vi "Panel Split Engine.vi"() -> ()   [LabVIEW 2013]
uses:
  PanelRootNode.lvclass
  <vilib>/Utility/error.llb/DialogType.ctl
  share/QueueManager.llb/Destroy.vi
  share/QueueManager.llb/CreatQueue.vi
  share/QueueManager.llb/Remove.vi
  PanelLinkNode/PanelLinkNode.lvclass
  PanelDataNode/PanelDataNode.lvclass
panel:
  out "SelfNode*":refnum<data-value>
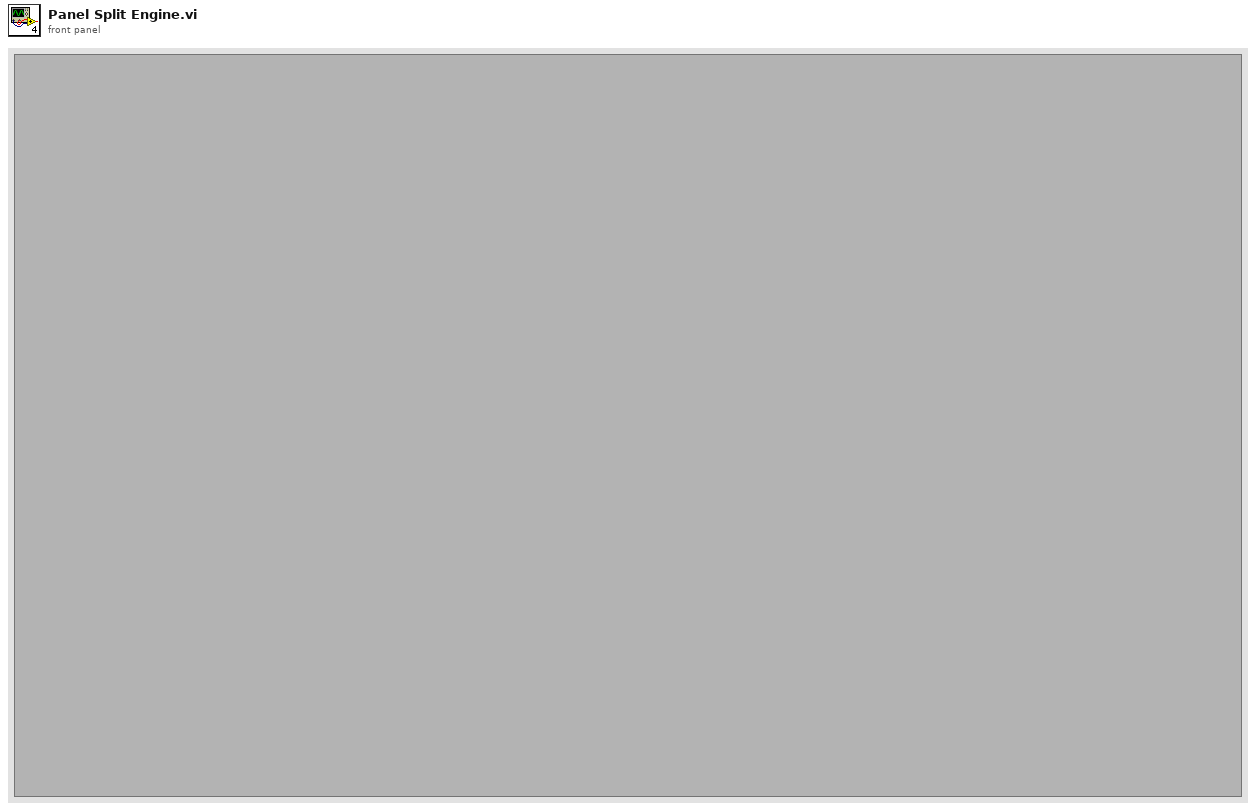
[diagram p1: front panel]
types:
  T1 = cluster{"error":errorcluster, "Event":string, "Data":variant, "Q_Local":string, "RootNode*":refnum<data-value>, "Caller":string}
  T2 = typedef "DialogType.ctl" = u16
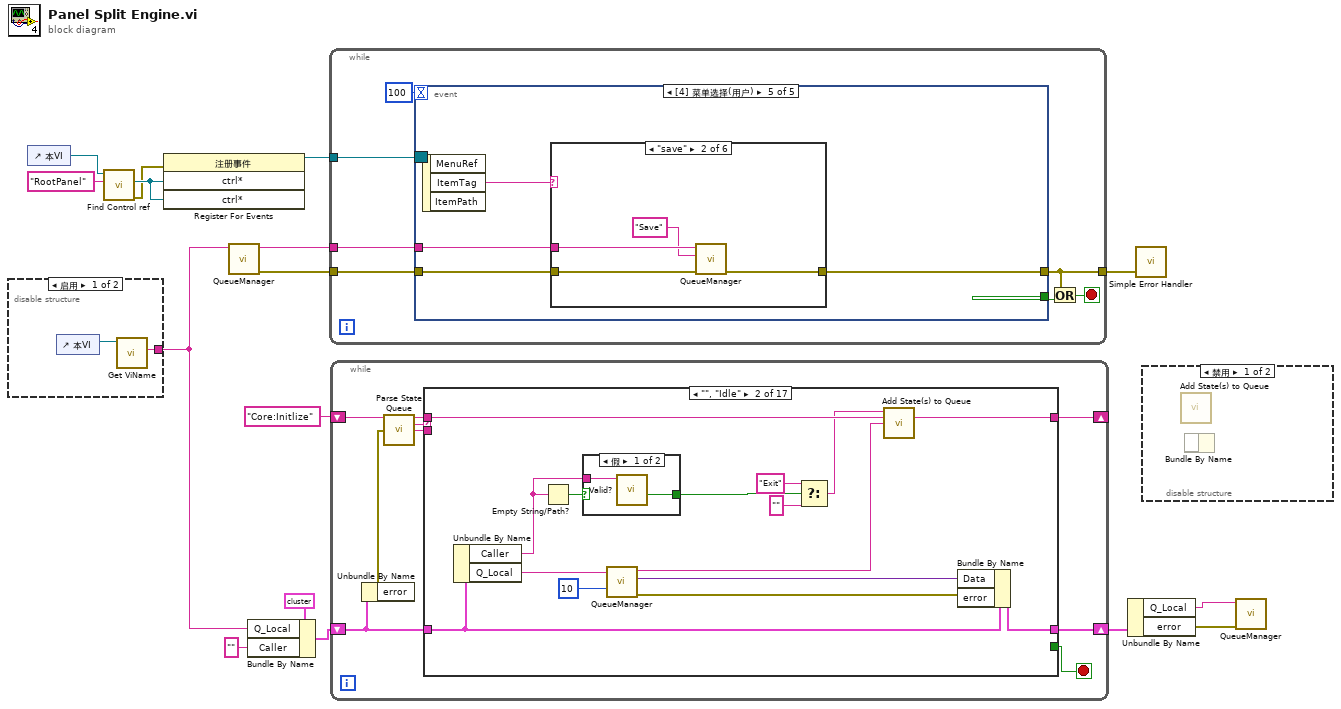
[diagram p0: block diagram]
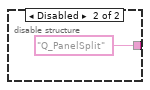
[diagram p2: hidden frame]
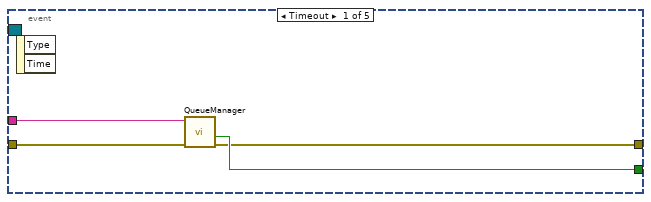
[diagram p4: hidden frame]
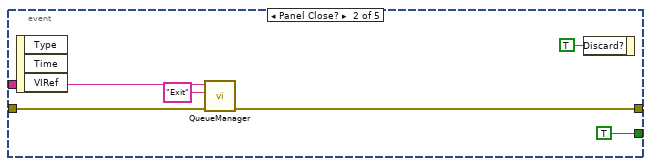
[diagram p5: hidden frame]
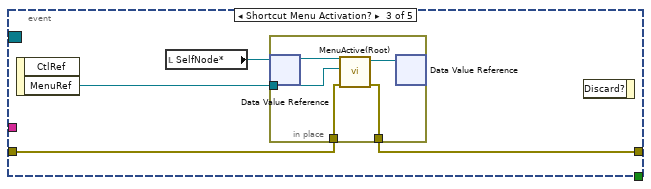
[diagram p6: hidden frame]
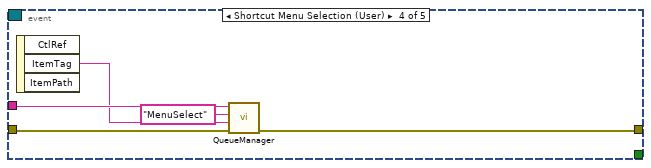
[diagram p7: hidden frame]
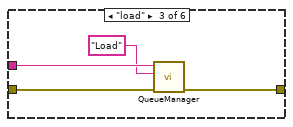
[diagram p9: hidden frame]
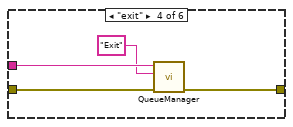
[diagram p10: hidden frame]
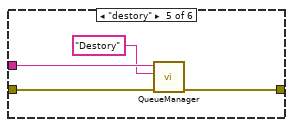
[diagram p11: hidden frame]
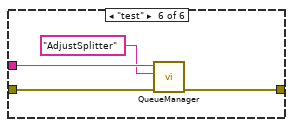
[diagram p12: hidden frame]
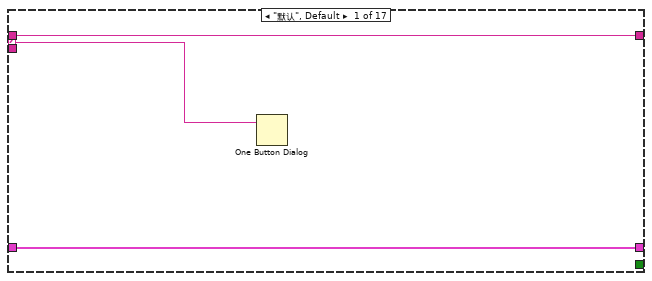
[diagram p13: hidden frame]
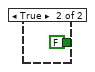
[diagram p14: hidden frame]
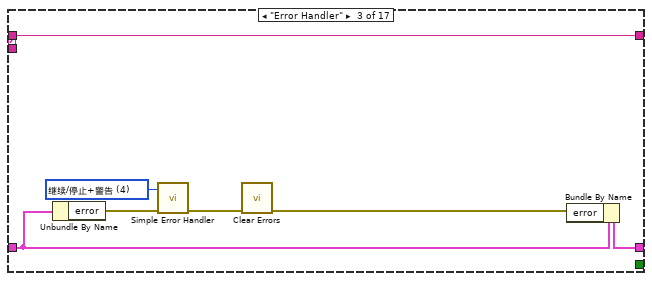
[diagram p15: hidden frame]
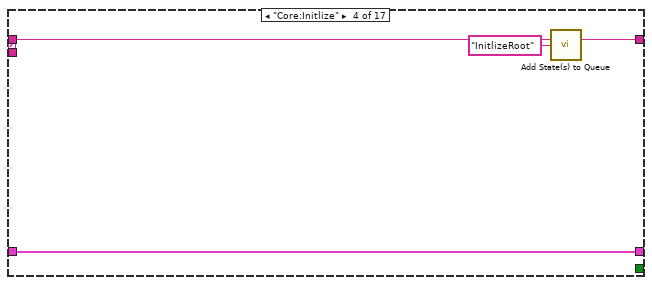
[diagram p16: hidden frame]
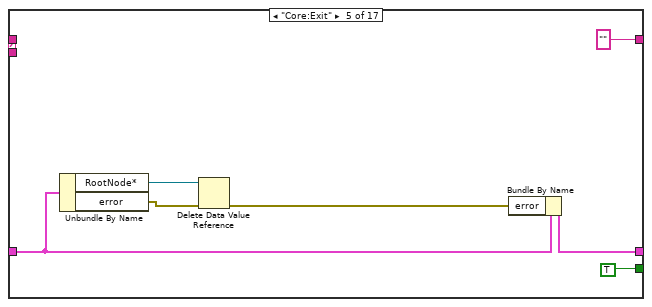
[diagram p17: hidden frame]
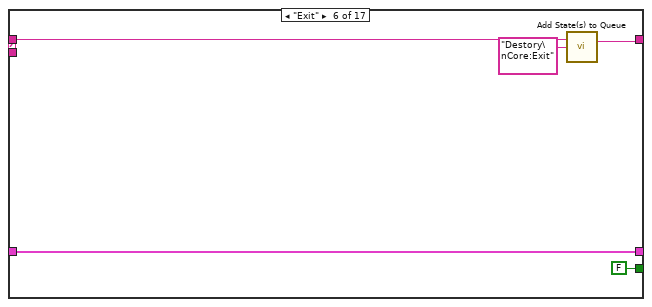
[diagram p18: hidden frame]
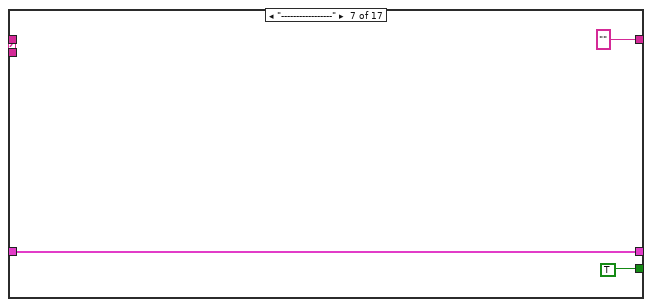
[diagram p19: hidden frame]
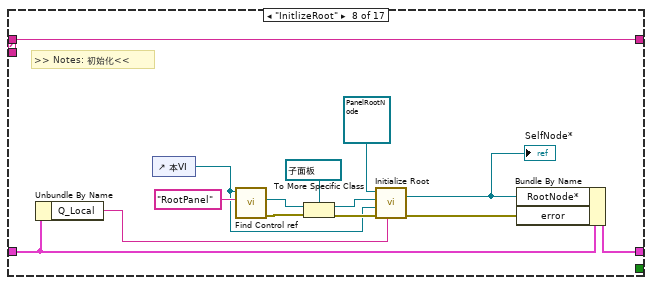
[diagram p20: hidden frame]
diagram:
  n1 = disable-structure shown="启用" {
    disable-tunnel: [w16 "Q_PanelSplit" ("QueueName")] -> w3
    frame Enabled {
      n2 = control-ref of="本VI"() -> (w17:refnum<vi>)
      n3 = call "Get ViName.vi"("VI*"=w17) -> ("VI Name"=w16:string)  [unwired: 8 in, 2 out]
    }
    frame Disabled {
    }
  }
  n4 = control-ref of="本VI"() -> (w7:refnum<vi>)
  n5 = call "Find Control ref.vi"("control name"="RootPanel", "panelvi*"=w7) -> ("error out"=w2:errorcluster, "ctrl*"=w5:refnum<vi>)  [unwired: 7 in, 1 out]
  n6 = register-events(error in=w2, w5, w5) -> (reference out=w4:refnum<event-registration>)  [unwired: 1 in, 1 out]
  n7 = call-poly "QueueManager.vi"("QueueName"=w3) -> ("error out"=w15:errorcluster)  [unwired: 10 in]
  n8 = Bundle By Name(cluster=T1 {"error"={"status"=FALSE, "code"=0, "source"=""}, "Event"="", "Data"=variant, "Q_Local"="", "RootNode*"=refnum, "Caller"=""} ("TmpData"), "Q_Local"=w3, "Caller"="") -> (w9:T1)
  n9 = while {
    tunnel: w15 -> [w24]
    tunnel: w3 -> [w25]
    tunnel: [w21] -> w11
    tunnel: w4 -> [w19]
    stop <- w22 stop-if-true
    n10 = event shown="[4] 菜单选择(用户)" {
      selector: w19 -> [_ _ _ _ _]
      dyn-events: _ -> [_ _ _ _ _]
      timeout: 100 -> [_ _ _ _ _]
      tunnel: [w27 TRUE _ _ _] -> w23
      tunnel: w25 -> [w29 w34 _ w49 w52]
      tunnel: w24 -> [w28 w33 w38 w48 w51]
      tunnel: [w26 w32 w39 w47 w50] -> w21
      event Timeout {
        n11 = event-data() -> ()  [unwired: 1 in, 2 out]
        n12 = call-poly "QueueManager.vi"("error in (no error)"=w28, "Queue Name(unamed)"=w29) -> ("error out"=w26:errorcluster, "Not Exist?"=w27:bool)  [unwired: 8 in]
      }
      event Panel Close? {
        n13 = event-data() -> ()  [unwired: 1 in, 3 out]
        n14 = call-poly "QueueManager.vi"("error in"=w33, "Event"="Exit", "QueueName"=w34) -> ("error out"=w32:errorcluster)  [unwired: 7 in, 1 out]
        n15 = event-data("Discard?"=TRUE ("放弃？")) -> ()  [unwired: 1 in, 1 out]
      }
      event Shortcut Menu Activation? {
        n16 = event-data() -> ("MenuRef"=w37:refnum<k9>)  [unwired: 1 in, 1 out]
        n17 = local read "SelfNode*"() -> (w36:refnum<data-value>)
        n18 = in-place {
          in-place-border: w37 -> [w42]
          in-place-border: w38 -> [w41]
          in-place-border: [w40] -> w39
          n19 = in-place-dvr #1(w36) -> (w44:refnum<class "PanelRootNode.lvclass">)  [unwired: 1 out]
          n20 = call "MenuActive(Root).vi"("error in (no error)"=w41, "菜单引用"=w42, "PanelDataNode 输入"=w44) -> ("error out"=w40:errorcluster, "PanelDataNode 输出"=w43:refnum<class "PanelRootNode.lvclass">)  [unwired: 7 in]
          n21 = in-place-dvr #1(w43) -> ()  [unwired: 2 out]
        }
        n22 = event-data() -> ()  [unwired: 2 in, 1 out]
      }
      event Shortcut Menu Selection (User) {
        n23 = event-data() -> ("ItemTag"=w46:string)  [unwired: 1 in, 2 out]
        n24 = call-poly "QueueManager.vi"("error in"=w48, "Data"=w46, "Event"="MenuSelect", "QueueName"=w49) -> ("error out"=w47:errorcluster)  [unwired: 6 in, 1 out]
      }
      event Menu Selection (User) {
        n25 = event-data() -> ("ItemTag"=w53:string)  [unwired: 1 in, 2 out]
        n26 = case shown="\"save\"" w53 {
          tunnel: w52 -> [_ w58 w62 w66 w70 w74]
          tunnel: w51 -> [w54 w56 w60 w64 w68 w72]
          tunnel: [w54 w55 w59 w63 w67 w71] -> w50
          frame "假", Default {
          }
          frame "save" {
            n27 = call-poly "QueueManager.vi"("error in"=w56, "Event"="Save", "QueueName"=w58) -> ("error out"=w55:errorcluster)  [unwired: 7 in, 1 out]
          }
          frame "load" {
            n28 = call-poly "QueueManager.vi"("error in"=w60, "Event"="Load", "QueueName"=w62) -> ("error out"=w59:errorcluster)  [unwired: 7 in, 1 out]
          }
          frame "exit" {
            n29 = call-poly "QueueManager.vi"("error in"=w64, "Event"="Exit", "QueueName"=w66) -> ("error out"=w63:errorcluster)  [unwired: 7 in, 1 out]
          }
          frame "destory" {
            n30 = call-poly "QueueManager.vi"("error in"=w68, "Event"="Destory", "QueueName"=w70) -> ("error out"=w67:errorcluster)  [unwired: 7 in, 1 out]
          }
          frame "test" {
            n31 = call-poly "QueueManager.vi"("error in"=w72, "Event"="AdjustSplitter", "QueueName"=w74) -> ("error out"=w71:errorcluster)  [unwired: 7 in, 1 out]
          }
        }
      }
    }
    n32 = Or(x=w21, y=w23) -> (x .or. y?=w22:bool)
  }
  n33 = while {
    shift-right: [w76] -> w12
    shift-left: w9 -> [w77]
    shift-right: [w75] -> _
    shift-left: "Core:Initlize" -> [w83]
    stop <- w79 stop-if-true
    n34 = Unbundle By Name(w77) -> ("error"=w78:errorcluster)
    n35 = call "Parse State Queue.vi"("State Queue"=w83, "Error In (no error)"=w78) -> ("Remaining States"=w82:string, "Current State"=w81:string, "Arguments"=w80:string)  [unwired: 10 in, 1 out]
    n36 = case shown="\"\", \"Idle\"" w81 {
      selector: w81 -> [w84 _ _ _ _ _ _ _ _ _ _ _ _ _ _ _ _]
      tunnel: w82 -> [w85 w97 w111 w114 _ w127 _ w144 w150 w166 w176 w191 w201 w211 w221 w230 w245]
      tunnel: w80 -> [_ _ _ _ _ _ _ _ _ _ _ _ _ _ _ _ _]
      tunnel: [_ _ _ _ TRUE FALSE TRUE _ _ _ _ _ _ _ _ _ _] -> w79
      tunnel: w77 -> [w86 w94 w107 w115 w118 w124 w129 w132 w152 w164 w180 w190 w199 w209 w219 w228 w243]
      tunnel: [w86 w100 w106 w115 w117 w124 w129 w135 w151 w163 w179 w189 w198 w208 w218 w227 w242] -> w76
      tunnel: [w85 w96 w111 w113 "" ("Remaining States") w126 "" ("Remaining States") w144 w150 w166 w175 w191 w201 w211 w221 w230 w245] -> w75
      frame "默认", Default {
        n37 = One Button Dialog(message=w84) -> ()  [unwired: 1 in, 1 out]
      }
      frame "", "Idle" {
        n38 = Unbundle By Name(w94) -> ("Caller"=w88:string, "Q_Local"=w93:string)
        n39 = Empty String/Path?(string/path=w88) -> (empty?=w92:bool)
        n40 = case shown="假" w92 {
          tunnel: [w103 FALSE ("Not Exist?")] -> w91
          tunnel: w88 -> [w102 _]
          frame False {
            n41 = call "Valid?.vi"("Queue Name(unamed)"=w102) -> ("Not Exist?"=w103:bool)  [unwired: 9 in, 1 out]
          }
          frame True {
          }
        }
        n42 = call-poly "QueueManager.vi"("Time out(-1)"=10, "Queue Name"=w93) -> ("error out"=w101:errorcluster, "Data"=w99:variant, "Event"=w98:string)  [unwired: 6 in, 1 out]
        n43 = Select(t="Exit" ("Event"), s=w91, f="") -> (s? t:f=w87:string)
        n44 = call "Add State(s) to Queue.vi"("State(s) in Front (\"\")"=w87, "State(s) in (\"\")"=w97, "State(s) at Back (\"\")"=w98) -> ("States Out"=w96:string)  [unwired: 12 in]
        n45 = Bundle By Name(cluster=w94, "Data"=w99, "error"=w101) -> (w100:T1)
      }
      frame "Error Handler" {
        w105 = T2 4 items=["无对话框", "确定信息", "继续或停止信息", "确定信息＋警告", "继续/停止+警告"] ("type of dialog (OK msg:1)")
        n46 = Unbundle By Name(w107) -> ("error"=w108:errorcluster)
        n47 = call <vilib>:"Simple Error Handler.vi"("type of dialog (OK msg:1)"=w105, "error in (no error)"=w108) -> ("error out"=w109:errorcluster)  [unwired: 3 in, 4 out]
        n48 = call <vilib>:"Clear Errors.vi"("error in (no error)"=w109) -> ("error out"=w110:errorcluster)  [unwired: 6 in]
        n49 = Bundle By Name(cluster=w107, "error"=w110) -> (w106:T1)
      }
      frame "Core:Initlize" {
        n50 = call "Add State(s) to Queue.vi"("State(s) in (\"\")"=w114, "State(s) at Back (\"\")"="InitlizeRoot" ("State(s) at Back (\"\")")) -> ("States Out"=w113:string)  [unwired: 13 in]
      }
      frame "Core:Exit" {
        n51 = Unbundle By Name(w118) -> ("RootNode*"=w120:refnum<data-value>, "error"=w116:errorcluster)
        n52 = Delete Data Value Reference(data value reference=w120, error in=w116) -> (error out=w119:errorcluster)  [unwired: 1 out]
        n53 = Bundle By Name(cluster=w118, "error"=w119) -> (w117:T1)
      }
      frame "Exit" {
        n54 = call "Add State(s) to Queue.vi"("State(s) in (\"\")"=w127, "State(s) at Back (\"\")"="Destory\nCore:Exit" ("State(s) at Back (\"\")")) -> ("States Out"=w126:string)  [unwired: 13 in]
      }
      frame "-----------------" {
      }
      frame "InitlizeRoot" {
        # ">> Notes: 初始化<<"
        n55 = Unbundle By Name(w132) -> ("Q_Local"=w131:string)
        n56 = control-ref of="本VI"() -> (w133:refnum<vi>)
        n57 = call "Find Control ref.vi"("control name"="RootPanel", "panelvi*"=w133) -> ("error out"=w138:errorcluster, "ctrl*"=w142:refnum<vi>)  [unwired: 7 in, 1 out]
        n58 = To More Specific Class(target class=refnum<vi> refnum ("RootPanel"), reference=w142, error in=w138) -> (specific class reference=w140:refnum<vi>, error out=w137:errorcluster)
        n59 = call-dynamic "Initialize Root.vi"("RootQueueName"=w131, "error in (no error)"=w137, "CurrentVi*"=w133, "RootPanel*"=w140, "PanelRootNode 输入"=refnum<class "PanelRootNode.lvclass"> refnum ("PanelRootNode.lvclass")) -> ("error out"=w136:errorcluster, "SelfNode*"=w134:refnum<data-value>)  [unwired: 5 in]
        "SelfNode*" <- w134
        n60 = Bundle By Name(cluster=w132, "RootNode*"=w134, "error"=w136) -> (w135:T1)
      }
      frame "Save" {
        # ">> Notes: 保存分割结果<<"
        n61 = Unbundle By Name(w152) -> ("RootNode*"=w153:refnum<data-value>, "Data"=w148:variant)
        n62 = Variant To Data(type=path "" ("路径"), Variant=w148) -> (data=w146:path, error out=w145:errorcluster)  [unwired: 1 in]
        n63 = call <vilib>:"Clear Errors.vi"("error in (no error)"=w145) -> ()  [unwired: 6 in, 1 out]
        n64 = in-place {
          in-place-border: [w155] -> w149
          in-place-border: w146 -> [w154]
          n65 = in-place-dvr #2(w153) -> (w157:refnum<class "PanelRootNode.lvclass">)  [unwired: 1 out]
          n66 = call-dynamic "Save Xml.vi"("selected path"=w154, "PanelRootNode 输入"=w157) -> ("error out"=w155:errorcluster, "PanelRootNode 输出"=w156:refnum<class "PanelRootNode.lvclass">)  [unwired: 8 in]
          n67 = in-place-dvr #2(w156) -> ()  [unwired: 2 out]
        }
        n68 = Bundle By Name(cluster=w152, "error"=w149) -> (w151:T1)
      }
      frame "Load" {
        n69 = Unbundle By Name(w164) -> ("RootNode*"=w165:refnum<data-value>, "Data"=w159:variant)
        n70 = Variant To Data(type=path "" ("路径"), Variant=w159) -> (data=w158:path, error out=w160:errorcluster)  [unwired: 1 in]
        n71 = call <vilib>:"Clear Errors.vi"("error in (no error)"=w160) -> ()  [unwired: 6 in, 1 out]
        n72 = in-place {
          in-place-border: [w169] -> w162
          in-place-border: w158 -> [w167]
          n73 = in-place-dvr #3(w165) -> (w168:refnum<class "PanelRootNode.lvclass">)  [unwired: 1 out]
          n74 = call-dynamic "Load Xml.vi"("selected path"=w167, "PanelRootNode 输入"=w168) -> ("error out"=w169:errorcluster, "PanelRootNode 输出"=w170:refnum<class "PanelRootNode.lvclass">)  [unwired: 8 in]
          n75 = in-place-dvr #3(w170) -> ()  [unwired: 2 out]
        }
        n76 = Bundle By Name(cluster=w164, "error"=w162) -> (w163:T1)
      }
      frame "MenuSelect" {
        n77 = Unbundle By Name(w180) -> ("RootNode*"=w174:refnum<data-value>, "Data"=w178:variant)
        n78 = Variant To Data(type="", Variant=w178) -> (data=w173:string, error out=w172:errorcluster)  [unwired: 1 in]
        n79 = in-place {
          in-place-border: w173 -> [w183]
          in-place-border: w172 -> [w182]
          in-place-border: [w181] -> w171
          n80 = in-place-dvr #4(w174) -> (w185:refnum<class "PanelRootNode.lvclass">)  [unwired: 1 out]
          n81 = call-dynamic "MenuSelect.vi"("error in"=w182, "Tag"=w183, "PanelRootNode 输入"=w185) -> ("error out"=w181:errorcluster, "PanelRootNode 输出"=w184:refnum<class "PanelRootNode.lvclass">)  [unwired: 7 in]
          n82 = in-place-dvr #4(w184) -> ()  [unwired: 2 out]
        }
        n83 = Bundle By Name(cluster=w180, "error"=w171) -> (w179:T1)
        n84 = call "Add State(s) to Queue.vi"("State(s) in (\"\")"=w176) -> ("States Out"=w175:string)  [unwired: 14 in]
      }
      frame "Split" {
        n85 = Unbundle By Name(w190) -> ("RootNode*"=w188:refnum<data-value>, "Data"=w187:variant)
        n86 = in-place {
          in-place-border: w187 -> [w193]
          in-place-border: [w192] -> w186
          n87 = in-place-dvr #5(w188) -> (w195:refnum<class "PanelRootNode.lvclass">)  [unwired: 1 out]
          n88 = call-dynamic "Split.vi"("Data"=w193, "PanelRootNode 输入"=w195) -> ("error out"=w192:errorcluster, "PanelRootNode 输出"=w194:refnum<class "PanelRootNode.lvclass">)  [unwired: 8 in]
          n89 = in-place-dvr #5(w194) -> ()  [unwired: 2 out]
        }
        n90 = Bundle By Name(cluster=w190, "error"=w186) -> (w189:T1)
      }
      frame "Delete" {
        n91 = Unbundle By Name(w199) -> ("RootNode*"=w200:refnum<data-value>, "Data"=w197:variant)
        n92 = in-place {
          in-place-border: w197 -> [w203]
          in-place-border: [w202] -> w196
          n93 = in-place-dvr #6(w200) -> (w205:refnum<class "PanelRootNode.lvclass">)  [unwired: 1 out]
          n94 = call-dynamic "Delete.vi"("Data"=w203, "PanelRootNode 输入"=w205) -> ("error out"=w202:errorcluster, "PanelRootNode 输出"=w204:refnum<class "PanelRootNode.lvclass">)  [unwired: 8 in]
          n95 = in-place-dvr #6(w204) -> ()  [unwired: 2 out]
        }
        n96 = Bundle By Name(cluster=w199, "error"=w196) -> (w198:T1)
      }
      frame "Insert" {
        n97 = Unbundle By Name(w209) -> ("RootNode*"=w210:refnum<data-value>, "Data"=w206:variant)
        n98 = in-place {
          in-place-border: [w212] -> w207
          in-place-border: w206 -> [w213]
          n99 = in-place-dvr #7(w210) -> (w215:refnum<class "PanelRootNode.lvclass">)  [unwired: 1 out]
          n100 = call-dynamic "Insert.vi"("Data"=w213, "PanelRootNode 输入"=w215) -> ("error out"=w212:errorcluster, "PanelRootNode 输出"=w214:refnum<class "PanelRootNode.lvclass">)  [unwired: 8 in]
          n101 = in-place-dvr #7(w214) -> ()  [unwired: 2 out]
        }
        n102 = Bundle By Name(cluster=w209, "error"=w207) -> (w208:T1)
      }
      frame "Destory" {
        # ">> Notes: 销毁分割结果，回到最初状态<<"
        n103 = Unbundle By Name(w219) -> ("RootNode*"=w220:refnum<data-value>, "Data"=w217:variant)
        n104 = in-place {
          in-place-border: w217 -> [_]
          in-place-border: [w222] -> w216
          n105 = in-place-dvr #8(w220) -> (w224:refnum<class "PanelRootNode.lvclass">)  [unwired: 1 out]
          n106 = call-dynamic "Destory.vi"("PanelRootNode 输入"=w224) -> ("error out"=w222:errorcluster, "PanelRootNode 输出"=w223:refnum<class "PanelRootNode.lvclass">)  [unwired: 9 in]
          n107 = in-place-dvr #8(w223) -> ()  [unwired: 2 out]
        }
        n108 = Bundle By Name(cluster=w219, "error"=w216) -> (w218:T1)
      }
      frame "AdjustSplitter" {
        # ">> Notes: 均分面板<<"
        n109 = Unbundle By Name(w228) -> ("RootNode*"=w229:refnum<data-value>, "Data"=w226:variant)
        n110 = in-place {
          in-place-border: w226 -> [_]
          in-place-border: [w231] -> w225
          n111 = in-place-dvr #9(w229) -> (w233:refnum<class "PanelRootNode.lvclass">)  [unwired: 1 out]
          n112 = call "Adjust Splitter.vi"("PanelRootNode 输入"=w233) -> ("error out"=w231:errorcluster, "PanelRootNode 输出"=w232:refnum<class "PanelRootNode.lvclass">)  [unwired: 9 in]
          n113 = in-place-dvr #9(w232) -> ()  [unwired: 2 out]
        }
        n114 = Bundle By Name(cluster=w228, "error"=w225) -> (w227:T1)
      }
      frame "SendToAll" {
        # ">> Notes: 发送至所有面板中插入的VI线程，要求插入的VI使用的队列名是VI名称；<<"
        n115 = Unbundle By Name(w243) -> ("RootNode*"=w244:refnum<data-value>, "Data"=w240:variant, "error"=w234:errorcluster)
        n116 = Variant To Data(error in=w234, type=cluster{"Event":string, "Data":variant} {"Event"="", "Data"=variant}, Variant=w240) -> (data=w238:cluster{"Event":string, "Data":variant}, error out=w235:errorcluster)
        n117 = Unbundle By Name(w238) -> ("Event"=w237:string, "Data"=w236:variant)
        n118 = in-place {
          in-place-border: [w250] -> w241
          in-place-border: w237 -> [w249]
          in-place-border: w236 -> [w248]
          in-place-border: w235 -> [w247]
          n119 = in-place-dvr #10(w244) -> (w252:refnum<class "PanelRootNode.lvclass">)  [unwired: 1 out]
          n120 = call "SendToPanels.vi"("PanelNumber(-1)"=-1, "error in"=w247, "Data"=w248, "Event"=w249, "PanelRootNode 输入"=w252) -> ("error out"=w250:errorcluster, "PanelRootNode 输出"=w251:refnum<class "PanelRootNode.lvclass">)  [unwired: 5 in]
          n121 = in-place-dvr #10(w251) -> ()  [unwired: 2 out]
        }
        n122 = Bundle By Name(cluster=w243, "error"=w241) -> (w242:T1)
      }
    }
  }
  n123 = Unbundle By Name(w12) -> ("Q_Local"=w8:string, "error"=w13:errorcluster)
  n124 = call <vilib>:"Simple Error Handler.vi"("error in (no error)"=w11) -> ()  [unwired: 4 in, 5 out]
  n125 = disable-structure shown="禁用" {
    frame Disabled {
      n126 = call "Add State(s) to Queue.vi"() -> ()  [unwired: 15 in, 1 out]
      n127 = Bundle By Name() -> ()  [unwired: 2 in, 1 out]
    }
    frame Enabled {
    }
  }
  n128 = call-poly "QueueManager.vi"("error in (no error)"=w13, "QueeuName"=w8) -> ()  [unwired: 9 in, 1 out]
